vi "RegisterExt.vi"   [LabVIEW 2014]
uses:
  <vilib>/registry/registry.llb/Registry RtKey.ctl
  control/DEF-RegExt.ctl
  application.lvclass
panel:
  # "Register LabVIEW file Extensions...."
types:
  T1 = typedef "Registry RtKey.ctl" = enum32{"HKEY_CLASSES_ROOT", "HKEY_CURRENT_USER", "HKEY_LOCAL_MACHINE", "HKEY_USERS", "HKEY_PERFORMANCE_DATA", "HKEY_CURRENT_CONFIG", "HKEY_DYN_DATA"}
  T2 = typedef "application.lvclass/DEF-RegExt.ctl" = cluster{"First Run?":bool, "Ext":string[]}
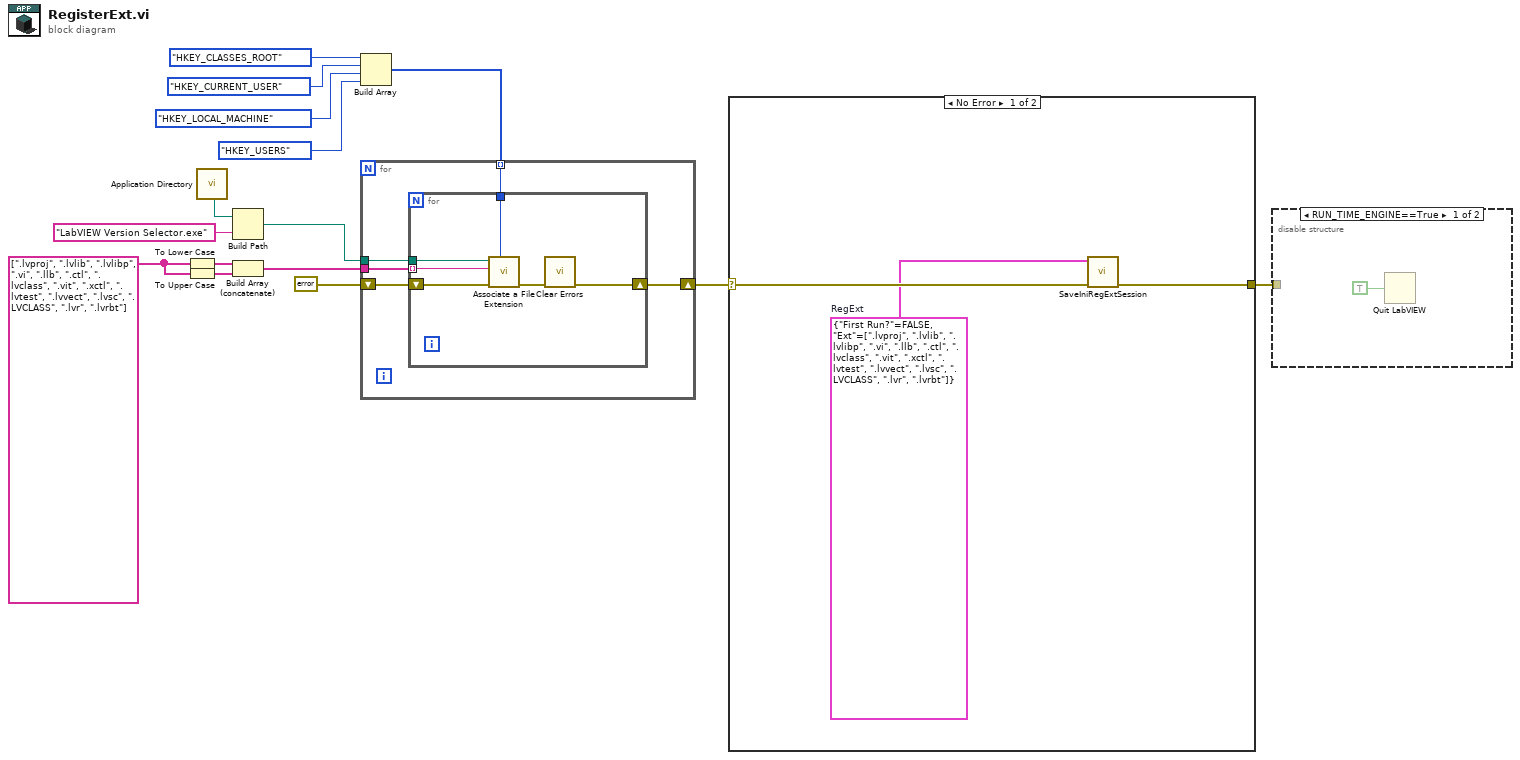
[diagram p0: block diagram]
diagram:
  w15 = string[] [".lvproj", ".lvlib", ".lvlibp", ".vi", ".llb", ".ctl", ".lvclass", ".vit", ".xctl", ".lvtest", ".lvvect", ".lvsc", ".LVCLASS", ".lvr", ".lvrbt"] ("Array")
  n1 = To Lower Case(string=w15) -> (all lower case string=w3:string[])
  n2 = To Upper Case(1:w15) -> (0:w14:string[])
  n3 = call <vilib>:"Application Directory.vi"() -> ("Application Directory"=w7:path)
  n4 = Build Path(base path=w7, name or relative path="LabVIEW Version Selector.exe") -> (appended path=w5:path)
  n5 = Build Array (concatenate)(w3, w14) -> (w13:string[])
  n6 = Build Array(Registry_RtKey."HKEY_CLASSES_ROOT" ("Root Key(HKLM)"), Registry_RtKey."HKEY_CURRENT_USER" ("Root Key(HKLM)"), Registry_RtKey."HKEY_LOCAL_MACHINE" ("Root Key(HKLM)"), Registry_RtKey."HKEY_USERS" ("Root Key(HKLM)")) -> (w8:T1[])
  n7 = for {
    tunnel: w13 -> [w19]
    tunnel: w8 -> [w20] mode=indexing
    tunnel: w5 -> [w18]
    shift-right: [w17] -> w2
    shift-left: errorcluster {"status"=FALSE, "code"=0, "source"=""} ("error out") -> [w16]
    n8 = for {
      tunnel: w20 -> [w26]
      tunnel: w19 -> [w25] mode=indexing
      tunnel: w18 -> [w24]
      shift-right: [w23] -> w17
      shift-left: w16 -> [w22]
      n9 = call "Associate a File Extension.vi"("Root Key(HKLM)"=w26, "error in (no error)"=w22, ".ext"=w25, "exe path"=w24) -> ("error out"=w21:errorcluster)  [unwired: 7 in]
      n10 = call <vilib>:"Clear Errors.vi"("error in (no error)"=w21) -> ("error out"=w23:errorcluster)  [unwired: 5 in, 1 out]
    }
  }
  n11 = case shown="No Error" w2 {
    selector: w2 -> [w29 w30]
    tunnel: [w28 w30] -> w1
    frame No Error {
      w27 = T2 {"First Run?"=FALSE, "Ext"=[".lvproj", ".lvlib", ".lvlibp", ".vi", ".llb", ".ctl", ".lvclass", ".vit", ".xctl", ".lvtest", ".lvvect", ".lvsc", ".LVCLASS", ".lvr", ".lvrbt"]}  # RegExt
      n12 = call "SaveIniRegExtSession.vi"("error in (no error)"=w29, "RegExt"=w27) -> ("error out"=w28:errorcluster)  [unwired: 9 in]
    }
    frame Error {
    }
  }
  n13 = disable-structure shown="RUN_TIME_ENGINE==True" {
    disable-tunnel: w1 -> [_ _]
    frame condition #0 {
      n14 = Quit LabVIEW(quit? (T)=TRUE) -> ()
    }
    frame condition #1 (active) {
    }
  }
